vi "StopPlayRslt.vi"(8 "error in (no error)":errorcluster, 11 "CameraTestingUI in":refnum<class "CameraTestingENI.lvclass">) -> (0 "error out":errorcluster, 3 "CameraTestingUI out":refnum<class "CameraTestingENI.lvclass">)   [LabVIEW 2020, in "CameraTestingProxy.lvlib" / "CameraTestingENI.lvclass"]
uses:
  CameraTestingENI.lvclass
  CameraTestingENI.lvclass/CameraTestingENI.ctl
  11315cb4-2454-4e75-9816-fc908c915b19.vi
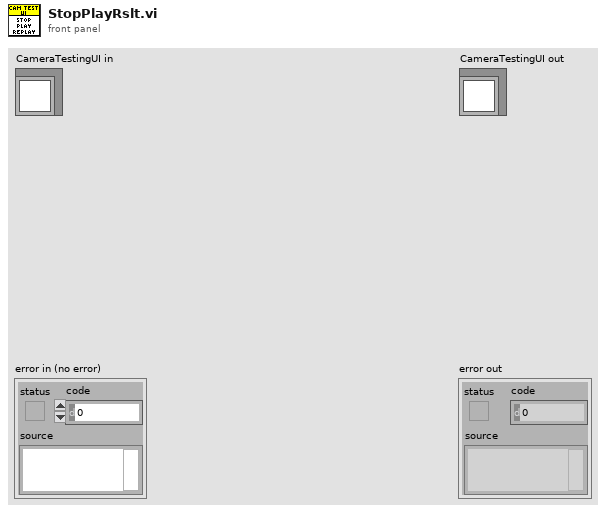
[diagram p1: front panel]
types:
  T1 = enum8{"Enabled", "Disabled", "Disabled and Grayed Out"}
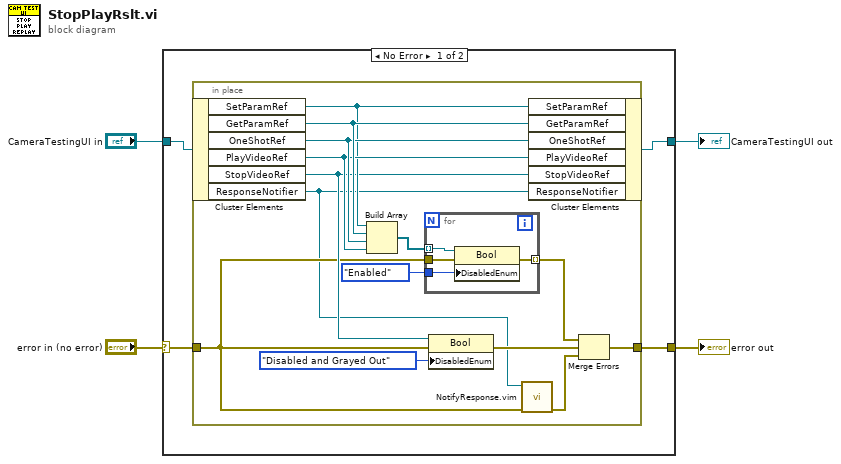
[diagram p0: block diagram]
diagram:
  n1 = case shown="No Error" "error in (no error)" {
    selector: "error in (no error)" -> [w7 w27]
    tunnel: "CameraTestingUI in" -> [w8 w28]
    tunnel: [w6 w28] -> w3
    tunnel: [w5 w27] -> w1
    frame No Error {
      n2 = in-place {
        in-place-border: w7 -> [w11]
        in-place-border: [w16] -> w5
        n3 = in-place-cluster #1(w8) -> ("SetParamRef"=w19:refnum<vi>, "GetParamRef"=w22:refnum<vi>, "OneShotRef"=w21:refnum<vi>, "PlayVideoRef"=w20:refnum<vi>, "StopVideoRef"=w15:refnum<vi>, "ResponseNotifier"=w9:refnum<notifier>)
        n4 = Build Array(w19, w22, w21, w20) -> (w18:refnum<vi>[])
        n5 = for {
          tunnel: w18 -> [w26] mode=indexing
          tunnel: w11 -> [w25]
          tunnel: [w24] -> w17 mode=indexing
          tunnel: T1."Enabled" ("Disabled") -> [w23]
          n6 = property class="Bool"(reference=w26, error in=w25, "DisabledEnum"=w23) -> (error out=w24:errorcluster)  [unwired: 1 out]
        }
        n7 = property class="Bool"(reference=w15, error in=w11, "DisabledEnum"=T1."Disabled and Grayed Out" ("Disabled")) -> (error out=w12:errorcluster)  [unwired: 1 out]
        n8 = call "NotifyResponse.vim"("error in (no error)"=w11, "ResponseNotifier"=w9) -> ("error out"=w10:errorcluster)  [unwired: 9 in]
        n9 = in-place-cluster #1("SetParamRef"=w19, "GetParamRef"=w22, "OneShotRef"=w21, "PlayVideoRef"=w20, "StopVideoRef"=w15, "ResponseNotifier"=w9) -> (w6:refnum<class "CameraTestingENI.lvclass">)
        n10 = Merge Errors(w17, w12, w10) -> (w16:errorcluster)
      }
    }
    frame Error {
    }
  }
  "error out" <- w1
  "CameraTestingUI out" <- w3
